vi "Neslab Serial Comms.vi"(0 "VISA resource name":refnum<visa-resource-name>, 1 "Addr MSB":u8 format="%02x", 2 "Addr LSB":u8=1 format="%02x", 5 "Command":T1(ring), 7 "Set Value":dbl format="%.2f", 11 "error in":errorcluster, 12 "Readback wait mS":u32=100, 13 "Report Cksm Err":bool=TRUE) -> (3 "write buffer(hex)":string, 4 "VISA out":refnum<visa-resource-name>, 6 "Numeric\nValue":dbl format="%.2f", 8 "String Value":string, 10 "Description":string, 14 "read buffer (hex)":string, 15 "error out":errorcluster)   [LabVIEW 2023]
panel:
  out "Checksum Fail":bool
  out "return count":u32
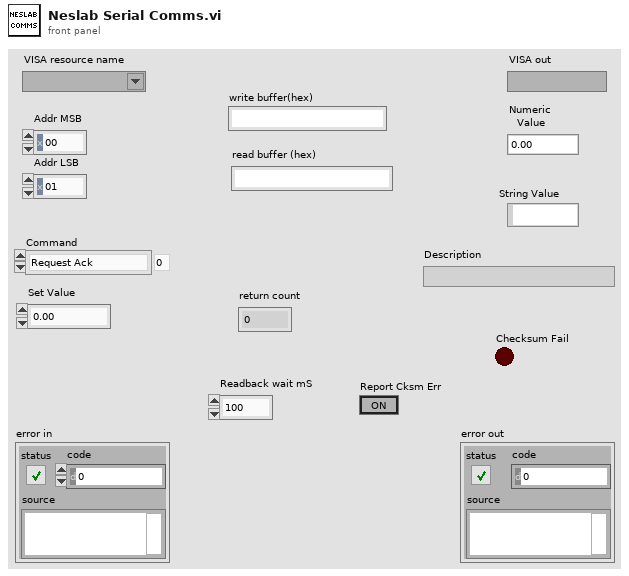
[diagram p1: front panel]
types:
  T1 = enum16{"Request Ack", "Set Setpoint", "Set Lo Limit", "Set Hi Limit", "Set Prop Band 0-99.9", "Set Integral 0-9.99", "Set Derivative 0-5.0", "Read Int Temp", "Read Ext Temp", "Read Setpoint", "Read Low Limit", "Read High Limit", "Read Prop Band", "Read Integral", "Read Derivative "}
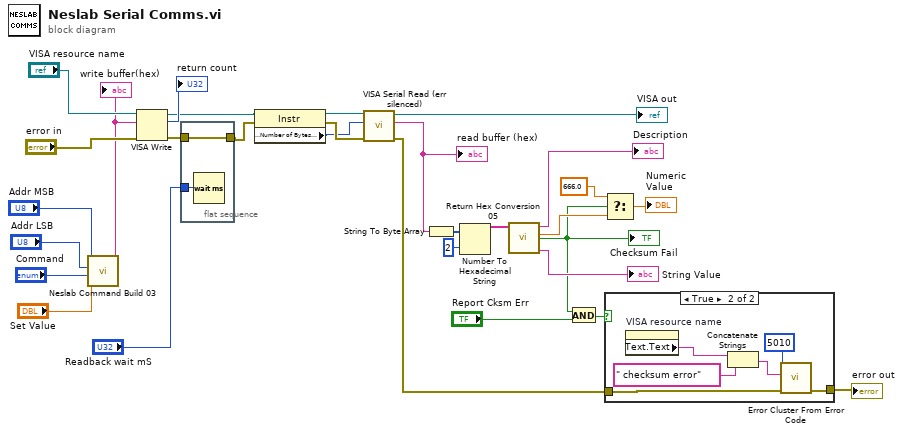
[diagram p0: block diagram]
diagram:
  n1 = call "Neslab Command Build 03.vi"("Set Value"="Set Value", "Command"="Command", "Addr LSB"="Addr LSB", "Addr MSB"="Addr MSB") -> ("Cmd Str"=w28:string)  [unwired: 3 in, 2 out]
  "write buffer(hex)" <- w28
  n2 = VISA Write(VISA resource name="VISA resource name", write buffer=w28, error in (no error)="error in") -> (VISA resource name out=w24:refnum<visa-resource-name>, return count=→"return count":u32, error out=w27:errorcluster)
  n3 = flat-sequence {
    tunnel: w27 -> [w32]
    tunnel: [w32] -> w21
    tunnel: "Readback wait mS" -> [w31]
    frame #0 {
      n4 = Wait (ms)(milliseconds to wait=w31) -> ()  [unwired: 1 out]
    }
  }
  n5 = property class="Instr"(reference=w24, error in=w21) -> (reference out=w23:refnum<visa-resource-name>, error out=w20:errorcluster, "Serial Settings:Number of Bytes at Serial Port"=w19:u32)
  n6 = call "VISA Serial Read (err silenced).vi"("error in"=w20, "byte count"=w19, "VISA resource name"=w23) -> ("error IO"=w11:errorcluster, "read buffer"=w18:string, "VISA resource name out"=→"VISA out":refnum<visa-resource-name>)  [unwired: 1 in, 1 out]
  "read buffer (hex)" <- w18
  n7 = String To Byte Array(string=w18) -> (unsigned byte array=w16:u8[])
  n8 = Number To Hexadecimal String(1:2, 2:w16) -> (0:w15:string[])
  n9 = call "Return Hex Conversion 05.VI"("Input Array"=w15) -> ("Value str"=→"String Value":string, "Vakue num"=w7:dbl, "Description"=→"Description":string, "Checksum Error"=w4:bool)  [unwired: 4 in, 1 out]
  "Checksum Fail" <- w4
  n10 = And(x=w4, y="Report Cksm Err") -> (x .and. y?=w9:bool)
  n11 = Select(t=666.0, s=w4, f=w7) -> (s? t:f=→"Numeric\nValue":dbl)
  n12 = case shown="True" w9 {
    tunnel: [w33 w38] -> w10
    tunnel: w11 -> [w33 w37]
    frame False {
    }
    frame True {
      n13 = property on="VISA resource name" class="VISAName"() -> ("Text.Text"=w35:string)  [unwired: 2 in, 2 out]
      n14 = Concatenate Strings(w35, " checksum error" ("error message (\"\")")) -> (w34:string)
      n15 = call <vilib>:"Error Cluster From Error Code.vi"("error in (no error)"=w37, "error message (\"\")"=w34, "error code (0)"=5010) -> ("error out"=w38:errorcluster)  [unwired: 6 in]
    }
  }
  "error out" <- w10
